vi "downsampling.vi"() -> ()   [LabVIEW 2014]
panel:
  out "波形图表":dynamicdata(graph)
  out "数值":dbl
  out "波形图":dynamicdata(graph)
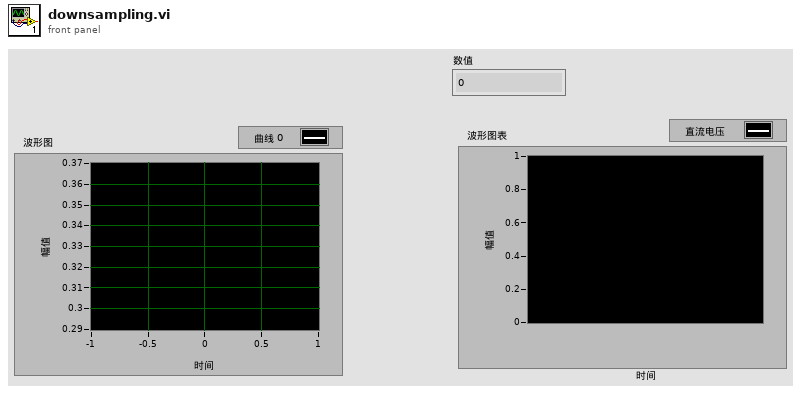
[diagram p1: front panel]
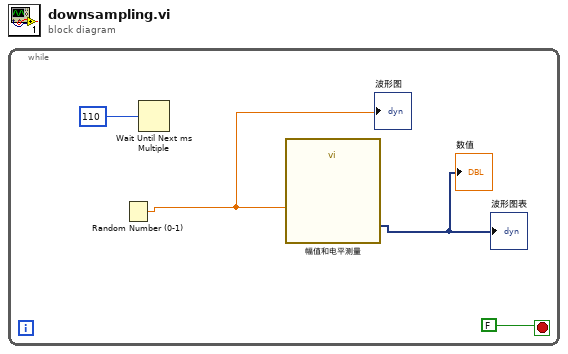
[diagram p0: block diagram]
diagram:
  n1 = while {
    stop <- FALSE stop-if-true
    n2 = Random Number (0-1)() -> (number: 0 to 1=w2:dbl)
    "波形图" <- w2
    n3 = Wait Until Next ms Multiple(millisecond multiple=110) -> ()  [unwired: 1 out]
    n4 = call "幅值和电平测量"("Signals"=w2) -> ("Mean (DC)"=→"数值" →"波形图表":dynamicdata)  [unwired: 13 in, 1 out]
  }
